vi "CANXNETWrite.vi"(8 "CAN1":T1[](array[typedef]) {"Data" format="%.0x"; "ArbitrationId" format="%.0x"; "Timestamp" format="%<%I:%M:%S%3u %p\n%m/%d/%Y>T"}, 9 "CAN0":T1[](array[typedef]) {"Data" format="%.0x"; "ArbitrationId" format="%.0x"; "Timestamp" format="%<%I:%M:%S%3u %p\n%m/%d/%Y>T"}, 11 "XNET":T2) -> (3 "XNET out":T2)   [LabVIEW 2017]
doc: "This example demonstrates frame streaming input using an NI-XNET Frame Input session. \n\nThis example can run against any output example, assuming you have a properly terminated CAN cable connected to two CAN ports.\n\nIf you have no database aliases on your system, the example automatically loads the nixnet_example database."
uses:
  <vilib>/nican/nican.llb/CanFrameTimed.ctl
  <vilib>/xnet/xnet.llb/XNET Frame CAN.ctl
  <vilib>/xnet/xnet.llb/XNET Frame Type CAN.ctl
  <vilib>/xnet/xnet.llb/XNET Write (Frame CAN).vi
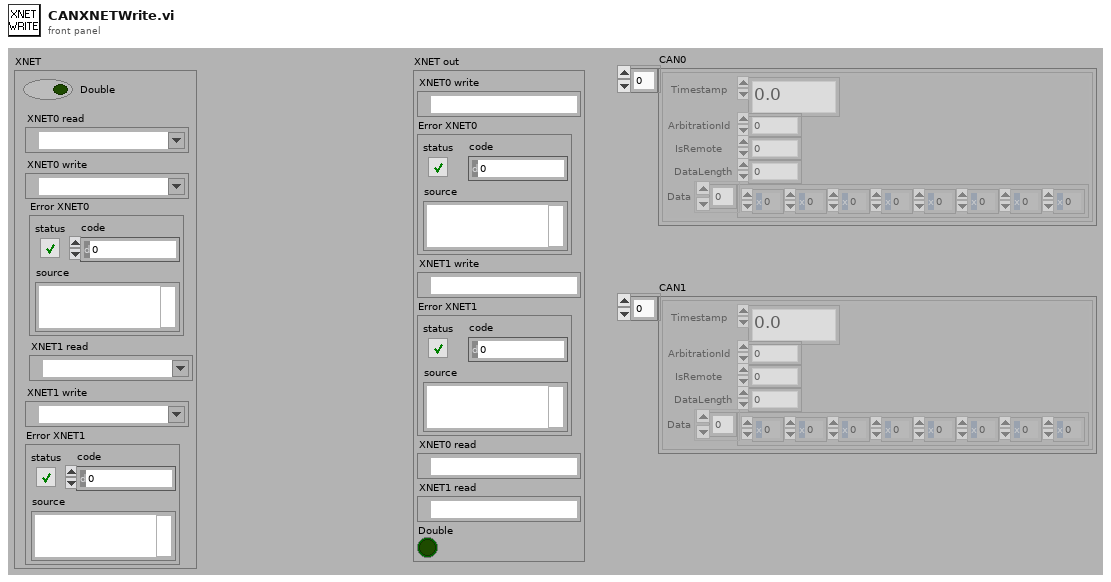
[diagram p1: front panel]
types:
  T1 = typedef "CanFrameTimed.ctl" = cluster{"Timestamp":dbl, "ArbitrationId":u32, "IsRemote":u8, "DataLength":u8, "Data":u8[]}
  T2 = cluster{"XNET0 write":refnum<k21>, "Error XNET0":errorcluster, "XNET1 write":refnum<k21>, "Error XNET1":errorcluster, "XNET0 read":refnum<k21>, "XNET1 read":refnum<k21>, "Double":bool}
  T3 = typedef "XNET Frame CAN.ctl" = cluster{"timestamp":timestamp, "payload":u8[], "identifier":u32, "type":T4, "extended?":bool, "echo?":bool}
  T4 = typedef "XNET Frame Type CAN.ctl" = u8
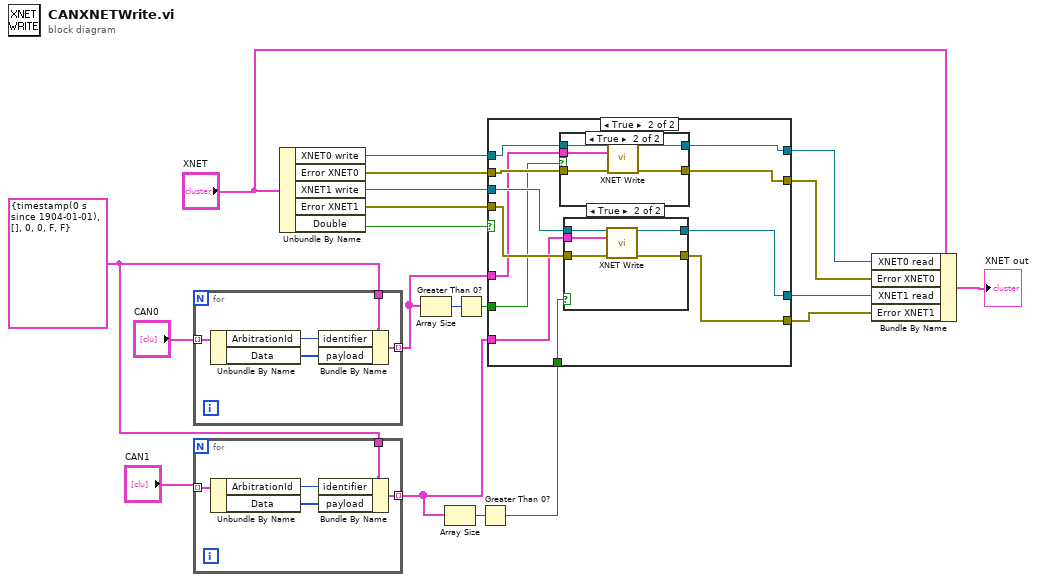
[diagram p0: block diagram]
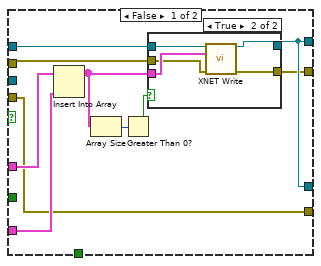
[diagram p2: hidden frame]
diagram:
  w9 = T3 {"timestamp"=timestamp(0 s since 1904-01-01), "payload"=[], "identifier"=0, "type"=0, "extended?"=FALSE, "echo?"=FALSE} ("CAN frame")
  n1 = for {
    tunnel: "CAN0" -> [w25] mode=indexing
    tunnel: w9 -> [w24]
    tunnel: [w21] -> w5 mode=indexing
    n2 = Unbundle By Name(w25) -> ("ArbitrationId"=w23:u32, "Data"=w22:u8[])
    n3 = Bundle By Name(cluster=w24, "identifier"=w23, "payload"=w22) -> (w21:T3)
  }
  n4 = for {
    tunnel: "CAN1" -> [w30] mode=indexing
    tunnel: w9 -> [w29]
    tunnel: [w26] -> w8 mode=indexing
    n5 = Unbundle By Name(w30) -> ("ArbitrationId"=w28:u32, "Data"=w27:u8[])
    n6 = Bundle By Name(cluster=w29, "identifier"=w28, "payload"=w27) -> (w26:T3)
  }
  n7 = Unbundle By Name("XNET") -> ("XNET0 write"=w2:refnum<k21>, "Error XNET0"=w1:errorcluster, "XNET1 write"=w20:refnum<k21>, "Error XNET1"=w19:errorcluster, "Double"=w16:bool)
  n8 = Array Size(array=w5) -> (size(s)=w6:i32)
  n9 = Array Size(array=w8) -> (size(s)=w7:i32)
  n10 = Greater Than 0?(x=w6) -> (x > 0?=w4:bool)
  n11 = Greater Than 0?(x=w7) -> (x > 0?=w3:bool)
  n12 = case shown="True" w16 {
    tunnel: w20 -> [_ w59]
    tunnel: w19 -> [w33 w58]
    tunnel: [w32 w55] -> w17
    tunnel: [w33 w56] -> w14
    tunnel: [w35 w54] -> w13
    tunnel: [w35 w57] -> w12
    tunnel: w8 -> [w39 w52]
    tunnel: w5 -> [w40 w51]
    tunnel: w1 -> [w31 w53]
    tunnel: w4 -> [_ w50]
    tunnel: w3 -> [_ w49]
    tunnel: w2 -> [w34 w48]
    frame False {
      n13 = Insert Into Array(array=w40, new element=w39) -> (w37:T3[])  [unwired: 1 in]
      n14 = Array Size(array=w37) -> (size(s)=w36:i32)
      n15 = Greater Than 0?(x=w36) -> (x > 0?=w38:bool)
      n16 = case shown="True" w38 {
        tunnel: w34 -> [w42 w47]
        tunnel: [w42 w46] -> w35
        tunnel: [w41 w45] -> w32
        tunnel: w37 -> [_ w44]
        tunnel: w31 -> [w41 w43]
        frame False {
        }
        frame True {
          n17 = call-poly <vilib>:"XNET Write.vi"("session in"=w47, "data"=w44, "error in (no error)"=w43) -> ("session out"=w46:refnum<k21>, "error out"=w45:errorcluster)  [unwired: 11 in]
        }
      }
    }
    frame True {
      n18 = case shown="True" w50 {
        tunnel: [w67 w73] -> w55
        tunnel: [w68 w72] -> w54
        tunnel: w48 -> [w68 w71]
        tunnel: w53 -> [w67 w70]
        tunnel: w51 -> [_ w69]
        frame False {
        }
        frame True {
          n19 = call-poly <vilib>:"XNET Write.vi"("session in"=w71, "data"=w69, "error in (no error)"=w70) -> ("session out"=w72:refnum<k21>, "error out"=w73:errorcluster)  [unwired: 11 in]
        }
      }
      n20 = case shown="True" w49 {
        tunnel: w59 -> [w61 w66]
        tunnel: w58 -> [w60 w65]
        tunnel: [w61 w64] -> w57
        tunnel: [w60 w63] -> w56
        tunnel: w52 -> [_ w62]
        frame False {
        }
        frame True {
          n21 = call-poly <vilib>:"XNET Write.vi"("session in"=w66, "data"=w62, "error in (no error)"=w65) -> ("session out"=w64:refnum<k21>, "error out"=w63:errorcluster)  [unwired: 11 in]
        }
      }
    }
  }
  n22 = Bundle By Name(cluster="XNET", "XNET0 read"=w13, "Error XNET0"=w17, "XNET1 read"=w12, "Error XNET1"=w14) -> (→"XNET out":T2)
